vi "GetPololuData.vi"() -> (0 "Right Board Voltage":dbl format="%#_4g", 1 "Right Board Temp":dbl format="%#_4g", 2 "Left Board Voltage":dbl, 3 "Left Board Temp":dbl format="%#_4g")   [LabVIEW 2017]
uses:
  <vilib>/myRIO/Instrument Drivers/Onboard IO/UART/typedef/VISA Configuration.ctl
  GlobalVarStop.vi
  <vilib>/Instr/_visa.llb/VISA Configure Serial Port (Instr).vi
  <vilib>/myRIO/Express VI/Onboard IO/UART/UART Express VI.xnode
  <vilib>/myRIO/Instrument Drivers/Onboard IO/UART/UART.lvlib
panel:
  out "error out":errorcluster
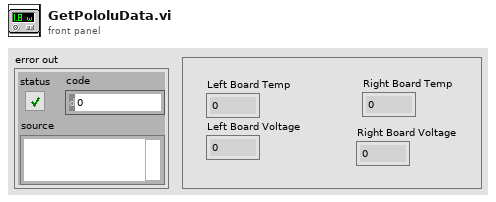
[diagram p1: front panel]
types:
  T1 = typedef "UART.lvlib/VISA Configuration.ctl" = cluster{"baud rate (9600)":u32, "data bits (8)":u16, "parity (0:none)":enum16{"None", "Odd", "Even", "Mark", "Space"}, "stop bits (10: 1 bit)":u16, "flow control (0:none)":u16, "termination char\n(0xA = '\\n' = LF) ":u8, "Enable Termination\nChar (T)":bool, "timeout (10sec)":u32}
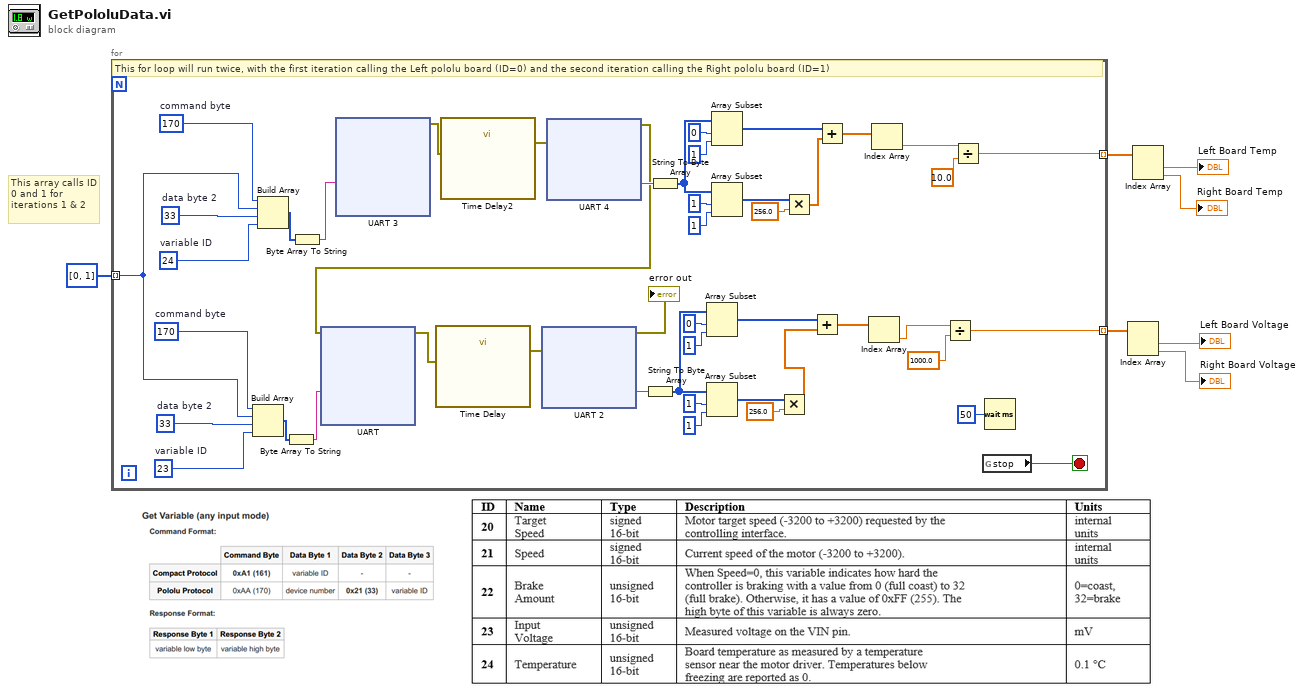
[diagram p0: block diagram]
diagram:
  # "This array calls ID 0 and 1 for iterations 1 & 2"
  n1 = for {
    tunnel: u8[] [0, 1] -> [w14] mode=indexing
    tunnel: [w13] -> w6 mode=indexing
    tunnel: [w12] -> w4 mode=indexing
    stop <- w8 stop-if-true
    w35 = u8 24  # variable ID
    w34 = u8 33  # data byte 2
    w31 = u8 170  # command byte
    w52 = u8 23  # variable ID
    w51 = u8 33  # data byte 2
    w48 = u8 170  # command byte
    # "This for loop will run twice, with the first iteration calling the Left pololu board (ID=0) and the second iteration calling the Right pololu board (ID=1)"
    n2 = Build Array(w48, w14, w51, w52) -> (w50:u8[])
    n3 = Build Array(w31, w14, w34, w35) -> (w33:u8[])
    n4 = Byte Array To String(unsigned byte array=w50) -> (string=w49:string)
    n5 = Byte Array To String(unsigned byte array=w33) -> (string=w32:string)
    n6 = xnode "UART 3"("Characters to Write"=w32) -> ("error out"=w36:errorcluster)  [unwired: 1 in, 1 out]
    n7 = call "Time Delay2"("error in (no error)"=w36) -> ("error out"=w37:errorcluster)  [unwired: 10 in]
    n8 = xnode "UART 4"("error in (no error)"=w37) -> ("Characters Read"=w30:string, "error out"=w11:errorcluster)
    n9 = xnode "UART"("Characters to Write"=w49, "error in (no error)"=w11) -> ("error out"=w53:errorcluster)  [unwired: 1 out]
    n10 = call "Time Delay"("error in (no error)"=w53) -> ("error out"=w54:errorcluster)  [unwired: 10 in]
    n11 = xnode "UART 2"("error in (no error)"=w54) -> ("Characters Read"=w47:string, "error out"=→"error out":errorcluster)
    n12 = String To Byte Array(string=w47) -> (unsigned byte array=w42:u8[])
    n13 = String To Byte Array(string=w30) -> (unsigned byte array=w25:u8[])
    n14 = Array Subset(array=w42, index=0, length=1) -> (w41:u8[])
    n15 = Array Subset(array=w42, index=1, length=1) -> (w39:u8[])
    n16 = Array Subset(array=w25, index=0, length=1) -> (w24:u8[])
    n17 = Array Subset(array=w25, index=1, length=1) -> (w22:u8[])
    n18 = Multiply(x=w39, y=256.0) -> (x*y=w19:dbl[])
    n19 = Multiply(x=w22, y=256.0) -> (x*y=w21:dbl[])
    n20 = Add(x=w41, y=w19) -> (x+y=w16:dbl[])
    n21 = Add(x=w24, y=w21) -> (x+y=w18:dbl[])
    n22 = Index Array(array=w16) -> (element=w15:dbl)  [unwired: 1 in]
    n23 = Index Array(array=w18) -> (element=w17:dbl)  [unwired: 1 in]
    n24 = Divide(x=w15, y=1000.0) -> (x/y=w12:dbl)
    n25 = Divide(x=w17, y=10.0) -> (x/y=w13:dbl)
    n26 = global read "GlobalVarStop.vi" "stop"() -> (w8:bool)
    n27 = Wait (ms)(milliseconds to wait=u32 50) -> ()  [unwired: 1 out]
  }
  n28 = Index Array(array=w4) -> (element #1=→"Left Board Voltage":dbl, element #2=→"Right Board Voltage":dbl)  [unwired: 2 in]
  n29 = Index Array(array=w6) -> (element #1=→"Left Board Temp":dbl, element #2=→"Right Board Temp":dbl)  [unwired: 2 in]
